vi "Agilent 364xA (GPIB,Serial) RT Driver VI.vi"(6 "Device Clock":string, 9 "Device Inputs FIFO":refnum<k33>, 10 "Device Outputs FIFO":refnum<k33>, 11 "Device Reference":T1 format="%.0x") -> ()   [LabVIEW 2010, in "Agilent 364xA (GPIB,Serial) Custom Device.lvlib"]
uses:
  Agilent 364xA (GPIB,Serial) Custom Device.lvlib
  <vilib>/NI VeriStand/Custom Device API/Custom Device Item Ref.ctl
  <vilib>/NI VeriStand/Custom Device API/Custom Device Channel Type.ctl
  <vilib>/Utility/error.llb/Simple Error Handler.vi
  <vilib>/NI Veristand/Custom Device API/Custom Device API.lvlib
  <vilib>/NI Veristand/Custom Device Tools/Custom Device Utility Library/Custom Device Utility Library.lvlib
panel:
  in  "Status Notifier":refnum<notifier>
  # "Custom Device Template\nv1.0"
  # "Use this template as a starting point for creating a custom device code module. The input controls shown here are specially named controls that the system will use to provide the device loop with data. The controls are not required for the device loop to run. For instance, if the device doesn't produce any output data, then you don't need the Device Outputs FIFO control. If you do use these controls, however, they need to have these exact names to be functional."
  # "The optional status notifier element is used to notify the RT engine of the last state of the custom device, and to indicate the device has completed execution. If this control is not used, a default No Error value is returned to the system when the device finishes execution.\n\nNote: This error state is not checked until the system shuts down. Use an output status channel to send more immediate status values to the system."
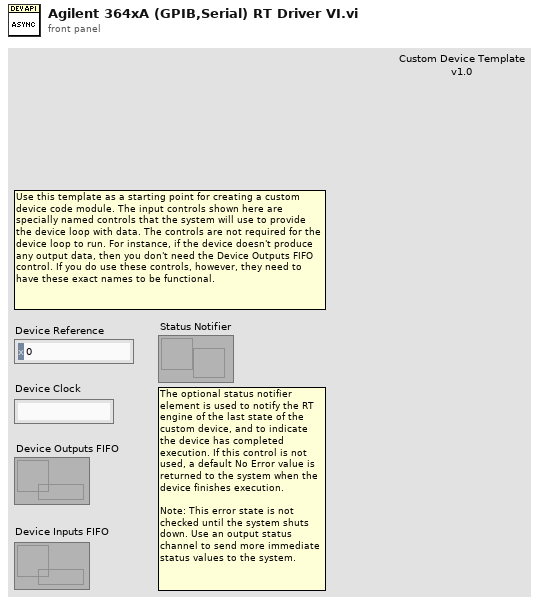
[diagram p1: front panel]
types:
  T1 = typedef "Custom Device API.lvlib/Custom Device Item Ref.ctl" = u64
  T2 = typedef "Custom Device API.lvlib/Custom Device Channel Type.ctl" = enum16{"Input", "Output"}
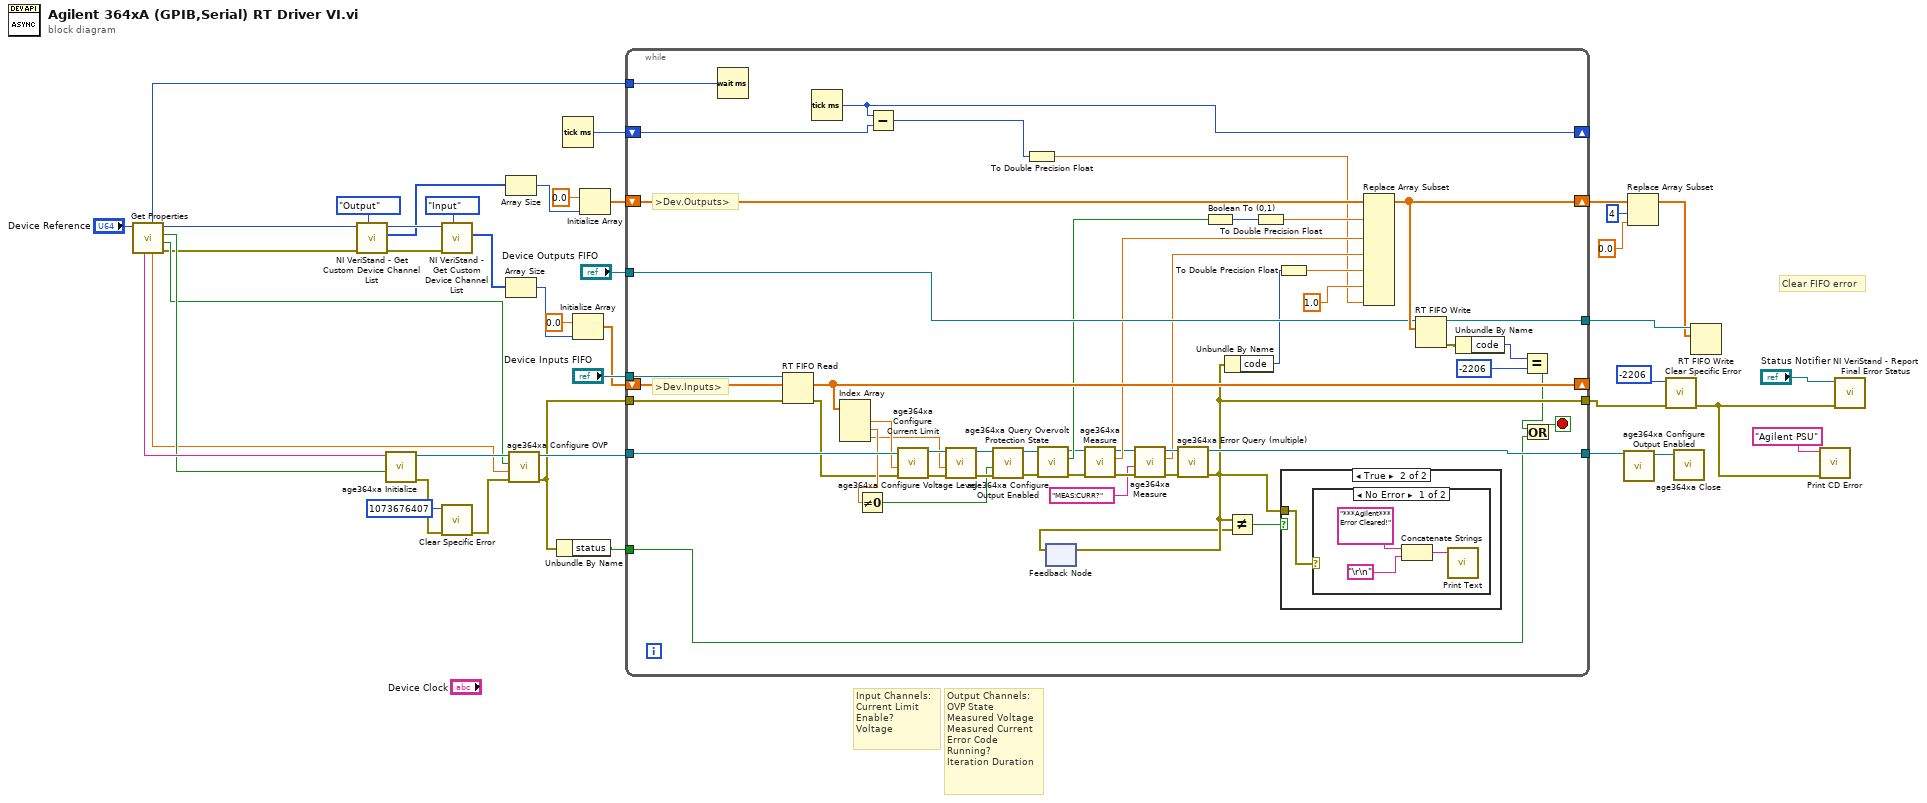
[diagram p0: block diagram]
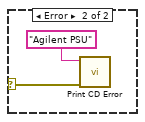
[diagram p3: hidden frame]
diagram:
  # "Clear FIFO error"
  # "Output Channels:\nOVP State\nMeasured Voltage\nMeasured Current\nError Code\nRunning?\nIteration Duration"
  # "Input Channels:\nCurrent Limit\nEnable?\nVoltage"
  n1 = call "Get Properties.vi"("Device Reference In"="Device Reference") -> ("error out"=w4:errorcluster, "Enable OVP"=w11:bool, "ID Query?"=w12:bool, "Device Reference Out"=w3:T1, "Voltage Limit"=w10:dbl, "Update Rate"=w2:u16, "VISA Resource Name"=w13:string)  [unwired: 4 in]
  n2 = call <vilib>:"NI VeriStand - Get Custom Device Channel List.vi"("Channel Type"=Custom_Device_Channel_Type."Output", "error in (no error)"=w4, "Device Ref in"=w3) -> ("error out"=w34:errorcluster, "Specified Channel Ref List"=w26:T1[], "Device Ref out"=w35:T1)  [unwired: 6 out]
  n3 = call <instrlib>:"age364xa Initialize.vi"("ID Query (T: Query)"=w12, "Instrument Resource Name"=w13) -> ("error out"=w7:errorcluster, "dup VISA session"=w16:refnum<visa-resource-name>)  [unwired: 8 in]
  n4 = call <vilib>:"NI VeriStand - Get Custom Device Channel List.vi"("Channel Type"=Custom_Device_Channel_Type."Input", "error in (no error)"=w34, "Device Ref in"=w35) -> ("Specified Channel Ref List"=w31:T1[])  [unwired: 8 out]
  n5 = call "Clear Specific Error.vi"("error in (no error)"=w7, "code"=1073676407) -> ("error out"=w6:errorcluster)  [unwired: 9 in]
  n6 = Array Size(array=w26) -> (size(s)=w32:i32)
  n7 = Array Size(array=w31) -> (size(s)=w30:i32)
  n8 = call <instrlib>:"age364xa Configure OVP.vi"("error in (no error)"=w6, "Limit (22.0 Volts)"=w10, "OVP Enabled (T: On)"=w11, "VISA session"=w16) -> ("error out"=w14:errorcluster, "dup VISA session"=w15:refnum<visa-resource-name>)  [unwired: 6 in]
  n9 = Unbundle By Name(w14) -> ("status"=w22:bool)
  n10 = Tick Count (ms)() -> (millisecond timer value=w1:u32)
  n11 = Initialize Array(0.0 ("element"), w30) -> (w37:dbl[])
  n12 = Initialize Array(0.0 ("element"), w32) -> (w38:dbl[])
  n13 = while {
    shift-right: [w90] -> _
    shift-left: w37 -> [w91]
    shift-right: [w88] -> w20
    shift-left: w38 -> [w89]
    tunnel: "Device Outputs FIFO" -> [w87]
    tunnel: "Device Inputs FIFO" -> [w86]
    tunnel: w15 -> [w85]
    tunnel: [w84] -> w9
    tunnel: w14 -> [w92]
    tunnel: [w83] -> w25
    tunnel: w22 -> [w81]
    tunnel: [w80] -> w21
    tunnel: w2 -> [w50]
    shift-right: [w43] -> _
    shift-left: w1 -> [w45]
    stop <- w82 stop-if-true
    # ">Dev.Outputs>"
    # ">Dev.Inputs>"
    n14 = Wait (ms)(milliseconds to wait=w50) -> ()  [unwired: 1 out]
    n15 = RT FIFO Read(0:w86, 1:w91, 3:w92) -> (9:w90:dbl[], 11:w68:errorcluster)  [unwired: 4 out]
    n16 = Tick Count (ms)() -> (millisecond timer value=w43:u32)
    n17 = Index Array(array=w90) -> (element #1=w75:dbl, element #2=w79:dbl, element #3=w72:dbl)  [unwired: 3 in]
    n18 = Not Equal To 0?(x=w79) -> (x != 0?=w69:bool)
    n19 = Subtract(x=w43, y=w45) -> (x-y=w44:u32)
    n20 = call <instrlib>:"age364xa Configure Current Limit.vi"("error in (no error)"=w68, "Current Limit (0.0 Amps)"=w75, "VISA session"=w85) -> ("error out"=w74:errorcluster, "dup VISA session"=w73:refnum<visa-resource-name>)  [unwired: 7 in]
    n21 = call <instrlib>:"age364xa Configure Voltage Level.vi"("error in (no error)"=w74, "Level (0.0 Volts)"=w72, "VISA session"=w73) -> ("error out"=w71:errorcluster, "dup VISA session"=w70:refnum<visa-resource-name>)  [unwired: 7 in]
    n22 = call <instrlib>:"age364xa Configure Output Enabled.vi"("error in (no error)"=w71, "Output Enabled (F: Off)"=w69, "VISA session"=w70) -> ("error out"=w67:errorcluster, "dup VISA session"=w66:refnum<visa-resource-name>)  [unwired: 7 in]
    n23 = To Double Precision Float(number=w44) -> (double precision float=w51:dbl)
    n24 = call <instrlib>:"age364xa Query Overvolt Protection State.vi"("error in (no error)"=w67, "VISA session"=w66) -> ("error out"=w62:errorcluster, "Over Voltage Protection"=w65:bool, "dup VISA session"=w61:refnum<visa-resource-name>)  [unwired: 7 in]
    n25 = feedback #1() -> (w77:errorcluster)  [unwired: 1 in]
    n26 = call <instrlib>:"age364xa Measure.vi"("error in (no error)"=w62, "VISA session"=w61) -> ("error out"=w57:errorcluster, "Measurement"=w60:dbl, "dup VISA session"=w56:refnum<visa-resource-name>)  [unwired: 7 in]
    n27 = call <instrlib>:"age364xa Measure.vi"("error in (no error)"=w57, "Measurement Type (Voltage)"="MEAS:CURR?", "VISA session"=w56) -> ("error out"=w55:errorcluster, "Measurement"=w53:dbl, "dup VISA session"=w54:refnum<visa-resource-name>)  [unwired: 6 in]
    n28 = call <instrlib>:"age364xa Error Query (multiple).vi"("error in (no error)"=w55, "VISA session"=w54) -> ("error out"=w83:errorcluster, "dup VISA session"=w84:refnum<visa-resource-name>)  [unwired: 6 in, 2 out]
    n29 = feedback-in #1(w83) -> ()
    n30 = Boolean To (0,1)(Boolean=w65) -> (0, 1=w64:i16)
    n31 = Unbundle By Name(w83) -> ("code"=w78:i32)
    n32 = Not Equal?(x=w83, y=w77) -> (x != y?=w76:bool)
    n33 = To Double Precision Float(number=w64) -> (double precision float=w63:dbl)
    n34 = To Double Precision Float(number=w78) -> (double precision float=w58:dbl)
    n35 = case shown="True" w76 {
      tunnel: w83 -> [_ w93]
      frame False {
      }
      frame True {
        n36 = case shown="No Error" w93 {
          selector: w93 -> [_ w97]
          frame No Error {
            n37 = Concatenate Strings("***Agilent*** Error Cleared!" ("string"), "\r\n") -> (w94:string)
            n38 = call "Print Text.vi"("Message"=w94) -> ()  [unwired: 11 in]
          }
          frame Error {
            n39 = call "Print CD Error.vi"("error out"=w97, "Your code's public name"="Agilent PSU") -> ()  [unwired: 9 in]
          }
        }
      }
    }
    n40 = Replace Array Subset(array=w89, new element #1=w63, new element #2=w60, new element #3=w53, new element #4=w58, new element #5=1.0 ("new element/subarray"), new element #6=w51) -> (w88:dbl[])  [unwired: 6 in]
    n41 = RT FIFO Write(0:w87, 1:w88) -> (8:w80:refnum<k33>, 11:w49:errorcluster)  [unwired: 2 in, 3 out]
    n42 = Unbundle By Name(w49) -> ("code"=w48:i32)
    n43 = Equal?(x=w48, y=-2206) -> (x = y?=w46:bool)
    n44 = Or(x=w46, y=w81) -> (x .or. y?=w82:bool)
  }
  n45 = call <instrlib>:"age364xa Configure Output Enabled.vi"("VISA session"=w9) -> ("dup VISA session"=w8:refnum<visa-resource-name>)  [unwired: 9 in, 1 out]
  n46 = Replace Array Subset(array=w20, new element=0.0 ("new element/subarray"), index=4) -> (w19:dbl[])
  n47 = call "Clear Specific Error.vi"("error in (no error)"=w25, "code"=-2206 ("x")) -> ("error out"=w23:errorcluster)  [unwired: 9 in]
  n48 = call <instrlib>:"age364xa Close.vi"("VISA session"=w8) -> ()  [unwired: 10 in, 1 out]
  n49 = RT FIFO Write(0:w21, 1:w19) -> ()  [unwired: 2 in, 5 out]
  n50 = call "Print CD Error.vi"("error out"=w23, "Your code's public name"="Agilent PSU") -> ()  [unwired: 9 in]
  n51 = call <vilib>:"NI VeriStand - Report Final Error Status.vi"("error in (no error)"=w23, "Status Notifier"="Status Notifier") -> ()  [unwired: 1 in, 9 out]
